vi "setup_furnitures.vi"(8 "error in":errorcluster, 11 "furntures in":refnum<class "Furniture.lvclass">[](array[class])) -> (0 "error out":errorcluster, 1 "Array":string[](array[string]), 3 "furntures out":refnum<class "Furniture.lvclass">[](array[class]))   [LabVIEW 2021]
uses:
  Furniture/Furniture.lvclass
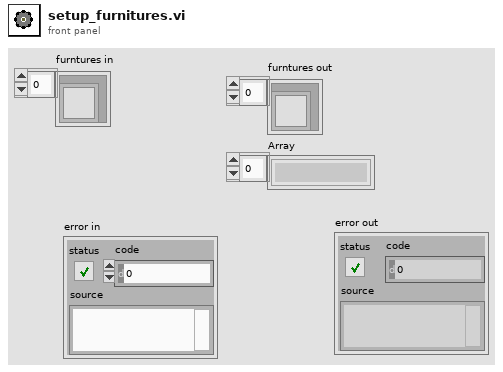
[diagram p1: front panel]
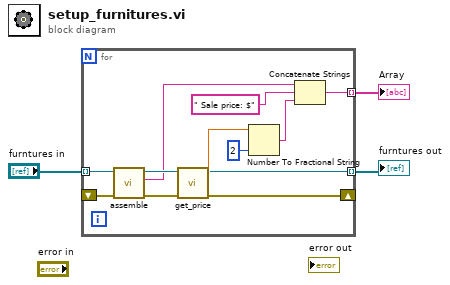
[diagram p0: block diagram]
diagram:
  n1 = for {
    tunnel: "furntures in" -> [w15] mode=indexing
    shift-right: [w11] -> _
    shift-left: _ -> [w13]
    tunnel: [w4] -> w2 mode=indexing
    tunnel: [w5] -> w1 mode=indexing
    n2 = call-dynamic "assemble.vi"("error in (no error)"=w13, "Furniture in"=w15) -> ("error out"=w12:errorcluster, "String"=w10:string, "Furniture out"=w14:refnum<class "Furniture.lvclass">)  [unwired: 7 in]
    n3 = call "get_price.vi"("error in (no error)"=w12, "Furniture in"=w14) -> ("error out"=w11:errorcluster, "price"=w8:dbl, "Furniture out"=w4:refnum<class "Furniture.lvclass">)  [unwired: 7 in]
    n4 = Number To Fractional String(number=w8, precision (6)=i16 2) -> (F-format string=w6:string)  [unwired: 2 in]
    n5 = Concatenate Strings(w10, " Sale price: $" ("string"), w6) -> (w5:string)
  }
  "furntures out" <- w2
  "Array" <- w1
